vi "Read configuration.vi"(8 "error in (no error)":errorcluster, 11 "Abstract Instrument in":refnum<class "Abstract Instrument.lvclass">) -> (0 "error out":errorcluster, 2 "CEF_configuration":refnum<class "CEF_serializable configuration.lvclass">, 3 "Abstract Instrument out":refnum<class "Abstract Instrument.lvclass">)   [LabVIEW 2025, in "Abstract Engine.lvlib" / "Abstract Instrument.lvclass"]
uses:
  Abstract Instrument.lvclass
  Users/Public/Documents/Sandia National Labs/TSS Plugin/CEF.lvlibp/serializable configuration/CEF_serializable configuration.lvclass
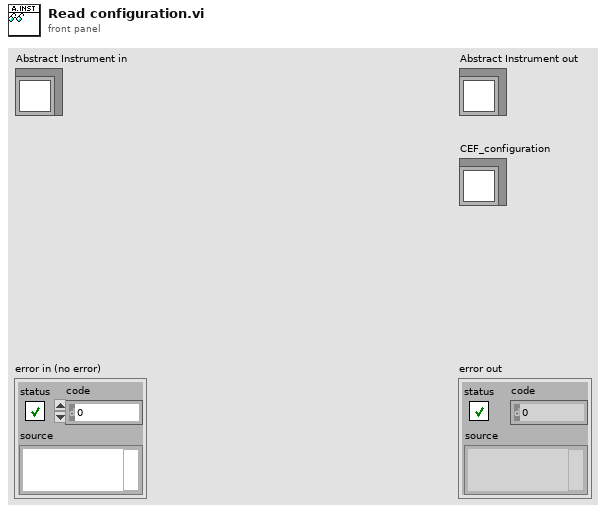
[diagram p1: front panel]
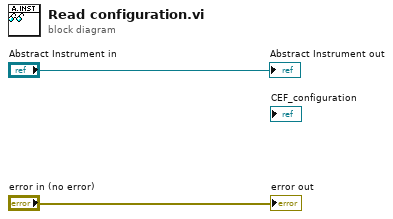
[diagram p0: block diagram]
diagram:
  "error out" <- "error in (no error)"
  "Abstract Instrument out" <- "Abstract Instrument in"
